vi "5.vi"() -> ()   [LabVIEW 2016]
panel:
  out "数组":dbl[](array[numeric])
  out "波形图 3":dbl[](graph)
  out "波形图 2":dbl[](graph)
  out "波形图":dbl[](graph)
  out "第三行":dbl[](array[numeric])
  out "第二行":dbl[](array[numeric])
  out "第一行":dbl[](array[numeric])
  out "总数组":dbl[][](array[numeric])
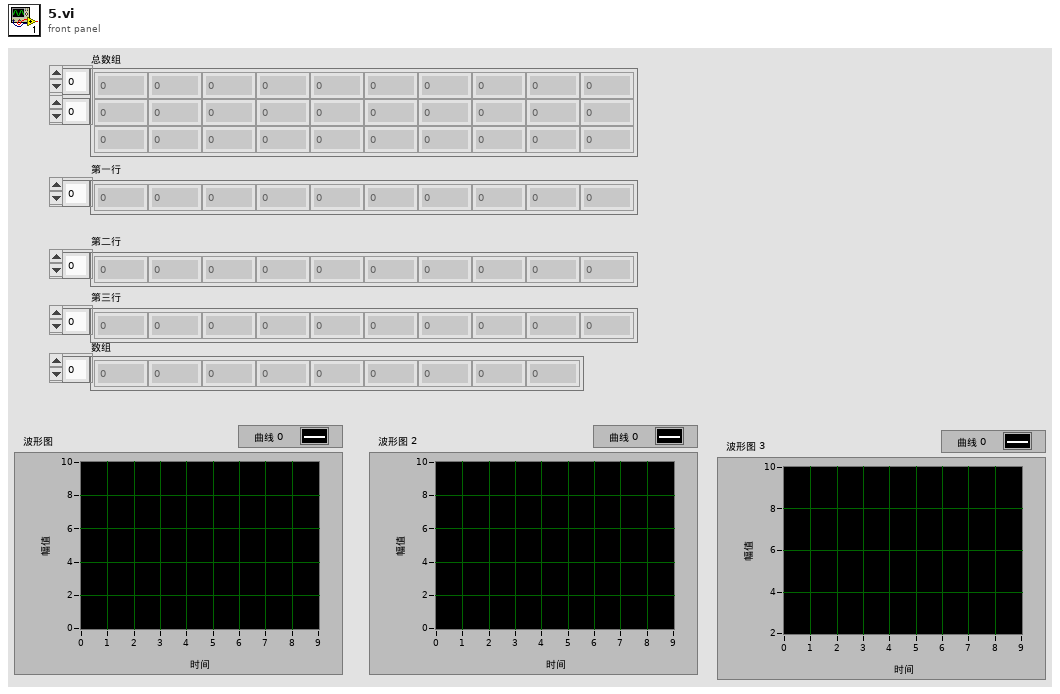
[diagram p1: front panel]
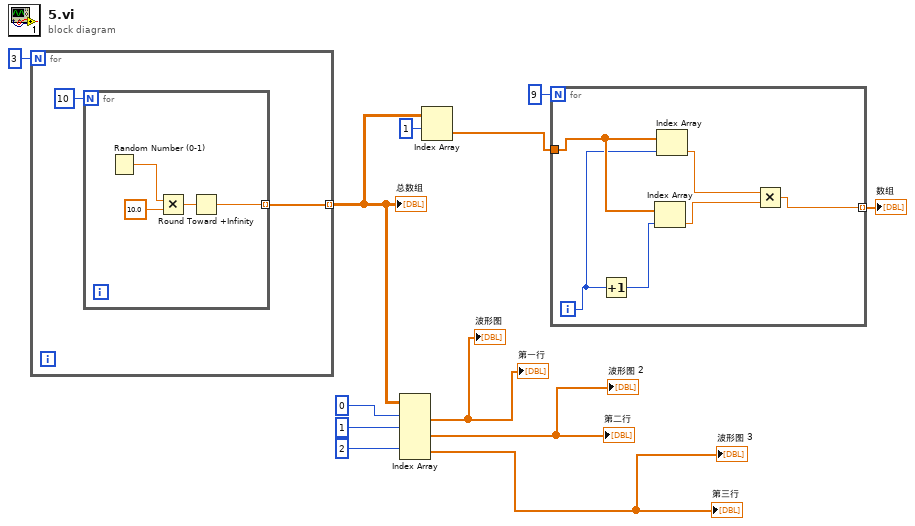
[diagram p0: block diagram]
diagram:
  n1 = for {
    N: 3 -> [_]
    tunnel: [w13] -> w4 mode=indexing
    n2 = for {
      N: 10 -> [_]
      tunnel: [w15] -> w13 mode=indexing
      n3 = Random Number (0-1)() -> (number: 0 to 1=w17:dbl)
      n4 = Multiply(x=w17, y=10.0) -> (x*y=w16:dbl)
      n5 = Round Toward +Infinity(x=w16) -> (ceil(x): smallest int >= x=w15:dbl)
    }
  }
  "总数组" <- w4
  n6 = Index Array(array=w4, index (row) #1=0 ("索引"), index (row) #2=1 ("索引"), index (row) #3=2 ("索引")) -> (element #1=→"第一行" →"波形图":dbl[], element #2=→"波形图 2" →"第二行":dbl[], element #3=→"波形图 3" →"第三行":dbl[])  [unwired: 3 in]
  n7 = Index Array(array=w4, index (row)=1 ("索引 (行)")) -> (element=w3:dbl[])  [unwired: 1 in]
  n8 = for {
    N: 9 -> [_]
    tunnel: w3 -> [w23]
    tunnel: [w20] -> w1 mode=indexing
    i -> [w21]
    n9 = Increment(x=w21) -> (x+1=w22:i32)
    n10 = Index Array(array=w23, index=w22) -> (element=w24:dbl)
    n11 = Index Array(array=w23, index=w21) -> (element=w19:dbl)
    n12 = Multiply(x=w19, y=w24) -> (x*y=w20:dbl)
  }
  "数组" <- w1
